vi "Measurement Logic.vi"() -> ()   [LabVIEW 2024, in "NIDCPowerSupplyAndSource.lvlib"]
uses:
  NIDCPowerSupplyAndSource.lvlib
  Measurement Configuration.ctl
  Measurement Results.ctl
  <vilib>/MeasurementLink/MeasurementLink Measurement Server/Measure Call Context/Measure Call Context.lvclass
  <vilib>/MeasurementLink/MeasurementLink Measurement Server/Measure Call Context/Reserve Sessions - 1Pin.vi
  <vilib>/MeasurementLink/MeasurementLink niDCPower/Get Connections - 1Pin 1Conn.vi
  <vilib>/MeasurementLink/MeasurementLink niDCPower/Initialize Sessions - 1Sess.vi
  <vilib>/MeasurementLink/MeasurementLink niDCPower/MeasurementLink niDCPower.lvlib
  <vilib>/MeasurementLink/MeasurementLink Session Management V1/Session Reservation/Session Reservation.lvclass
panel:
  out "measure call context out":refnum<class "Measure Call Context.lvclass">
  in  "measure call context in":refnum<class "Measure Call Context.lvclass">
  out "measurement results":T1
  in  "measurement configuration":T2
  out "error out":errorcluster
  in  "error in":errorcluster
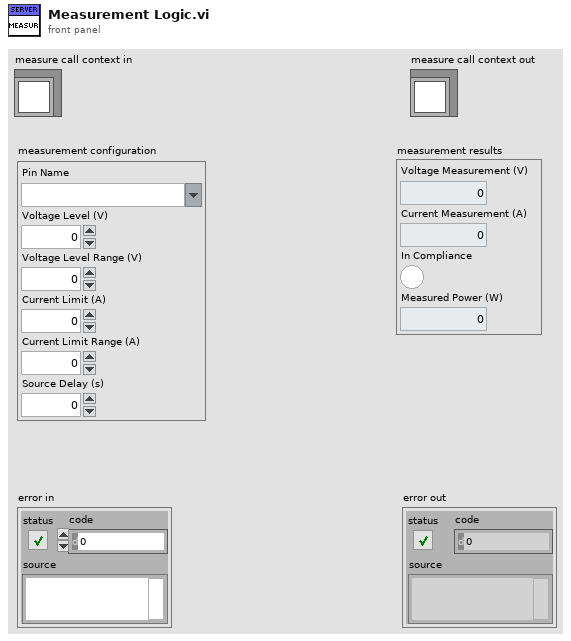
[diagram p1: front panel]
types:
  T1 = typedef "NIDCPowerSupplyAndSource.lvlib/Measurement Results.ctl" = cluster{"Voltage Measurement (V)":dbl, "Current Measurement (A)":dbl, "In Compliance":bool, "Measured Power (W)":dbl}
  T2 = typedef "NIDCPowerSupplyAndSource.lvlib/Measurement Configuration.ctl" = cluster{"Pin Name":string, "Voltage Level (V)":dbl, "Voltage Level Range (V)":dbl, "Current Limit (A)":dbl, "Current Limit Range (A)":dbl, "Source Delay (s)":dbl}
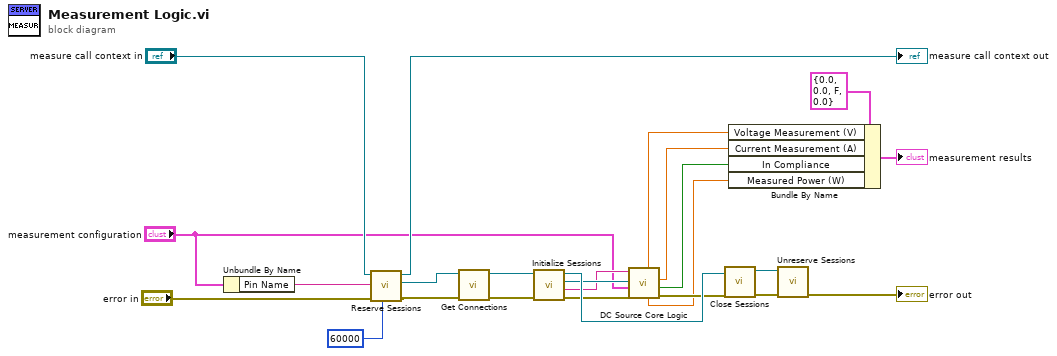
[diagram p0: block diagram]
diagram:
  n1 = Unbundle By Name("measurement configuration") -> ("Pin Name"=w22:string)
  n2 = call-poly <vilib>:"Reserve Sessions.vi"("timeout (ms)"=60000, "error in"="error in", "pin or relay name"=w22, "measurement context in"="measure call context in") -> ("error out"=w21:errorcluster, "session reservation out"=w17:refnum<class "Session Reservation.lvclass">, "measurement context out"=→"measure call context out":refnum<class "Measure Call Context.lvclass">)  [unwired: 5 in]
  n3 = call-poly <vilib>:"Get Connections.vi"("error in"=w21, "session reservation in"=w17) -> ("error out"=w24:errorcluster, "session reservation out"=w23:refnum<class "Session Reservation.lvclass">)  [unwired: 7 in, 1 out]
  n4 = call-poly <vilib>:"Initialize Sessions.vi"("error in"=w24, "session reservation in"=w23) -> ("error out"=w8:errorcluster, "channel list"=w10:string, "session"=w11:refnum<k15>, "session reservation out"=w12:refnum<class "Session Reservation.lvclass">)  [unwired: 6 in]
  n5 = call "DC Source Core Logic.vi"("error in"=w8, "measurement configuration"="measurement configuration", "instrument handle"=w11, "channel list"=w10) -> ("error out"=w7:errorcluster, "in compliance?"=w2:bool, "measured current"=w3:dbl, "calculated power"=w1:dbl, "measured voltage"=w4:dbl)  [unwired: 2 in, 1 out]
  n6 = call <vilib>:"Close Sessions.vi"("error in"=w7, "session reservation in"=w12) -> ("error out"=w16:errorcluster, "session reservation out"=w15:refnum<class "Session Reservation.lvclass">)  [unwired: 8 in]
  n7 = Bundle By Name(cluster=T1 {"Voltage Measurement (V)"=0.0, "Current Measurement (A)"=0.0, "In Compliance"=FALSE, "Measured Power (W)"=0.0} ("Measurement Results"), "Voltage Measurement (V)"=w4, "Current Measurement (A)"=w3, "In Compliance"=w2, "Measured Power (W)"=w1) -> (→"measurement results":T1)
  n8 = call <vilib>:"Unreserve Sessions.vi"("error in"=w16, "session reservation in"=w15) -> ("error out"=→"error out":errorcluster)  [unwired: 9 in]
